vi "CheckForErrors.vi"() -> ()   [LabVIEW 2019]
panel:
  out "Returned one parameter":dbl
  out "Errors":string
  out "Returned parameters":string[](array[string])
  in  "Parameters":string[](array[string])
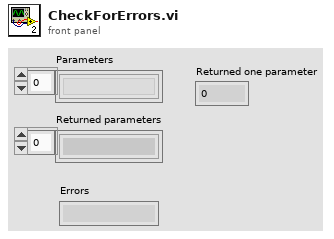
[diagram p1: front panel]
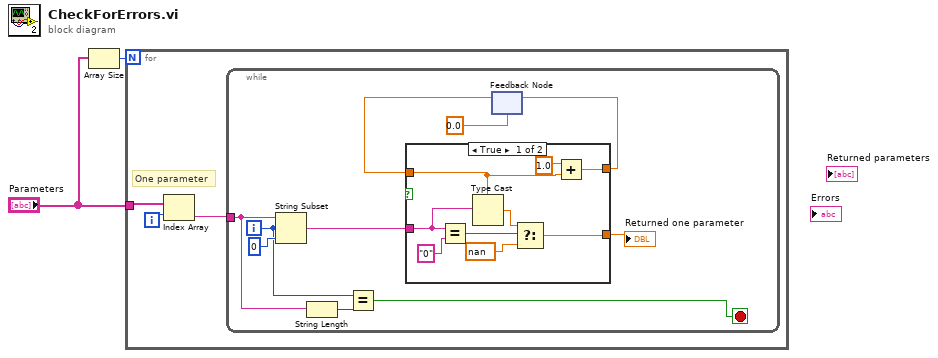
[diagram p0: block diagram]
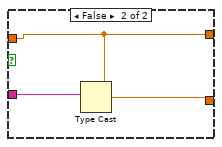
[diagram p2: hidden frame]
diagram:
  n1 = Array Size(array="Parameters") -> (size(s)=w2:i32)
  n2 = for {
    N: w2 -> [_]
    tunnel: "Parameters" -> [w5]
    i -> [w4]
    # "One parameter"
    n3 = Index Array(array=w5, index=w4) -> (element=w3:string)
    n4 = while {
      tunnel: w3 -> [w8]
      i -> [w7]
      stop <- w6 stop-if-true
      n5 = String Subset(string=w8, offset (0)=w7, length (rest)=0) -> (substring=w12:string)
      n6 = String Length(string=w8) -> (length=w9:i32)
      n7 = Equal?(x=w7, y=w9) -> (x = y?=w6:bool)
      n8 = feedback #1(0.0 ("x")) -> (w14:dbl)
      n9 = case shown="True" {
        selector: _ -> [_ _]
        tunnel: [w24 w26] -> w15
        tunnel: w14 -> [w16 w26]
        tunnel: w12 -> [w19 w27]
        tunnel: [w17 w25] -> w10
        frame True {
          n10 = Equal?(x=w19, y="0") -> (x = y?=w21:bool)
          n11 = Type Cast(type=w16, x=w19) -> (*(type *) &x=w18:dbl)
          n12 = Select(t=w18, s=w21, f=nan) -> (s? t:f=w17:dbl)
          n13 = Add(x=1.0, y=w16) -> (x+y=w24:dbl)
        }
        frame False {
          n14 = Type Cast(type=w26, x=w27) -> (*(type *) &x=w25:dbl)
        }
      }
      "Returned one parameter" <- w10
      n15 = feedback-in #1(w15) -> ()
    }
  }
